vi "Get Intermediate Result.vi"(8 "error in (no error)":errorcluster, 11 "AverageCollector1D in":refnum<class "AverageCollector1D.lvclass">) -> (0 "error out":errorcluster, 2 "AbstractData.lvclass":refnum<class "AbstractData.lvclass">, 3 "AverageCollector1D out":refnum<class "AverageCollector1D.lvclass">)   [LabVIEW 2014, in "AverageCollector1D.lvclass"]
uses:
  AverageCollector1D.lvclass
  Framework/Model/Data/AbstractData/AbstractData.lvclass
  Framework/Collector/AbstractCollector/AbstractCollector.lvclass/AbstractCollector.ctl
  Framework/Model/Data/Data1D/Data1D.lvclass
  Framework/Collector/AbstractCollector/AbstractCollector.lvclass
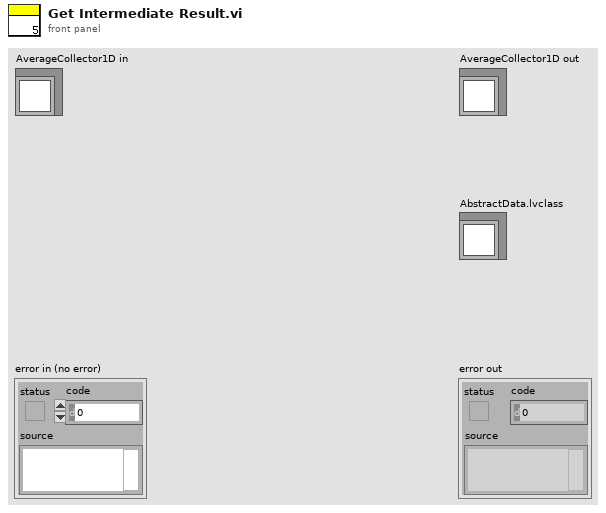
[diagram p1: front panel]
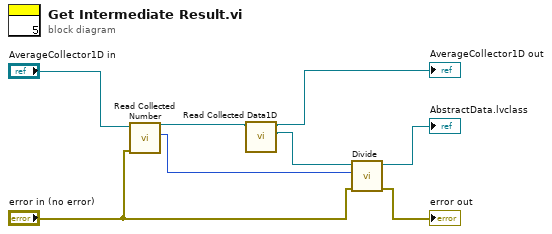
[diagram p0: block diagram]
diagram:
  n1 = call "Read Collected Number.vi"("error in (no error)"="error in (no error)", "AbstractCollector in"="AverageCollector1D in") -> ("collected"=w7:u32, "AbstractCollector out"=w4:refnum<class "AverageCollector1D.lvclass">)  [unwired: 7 in, 1 out]
  n2 = call-dynamic "Read Collected Data1D.vi"("AbstractCollector1D in"=w4) -> ("Collected Data"=w3:refnum<class "Data1D.lvclass">, "AbstractCollector1D out"=→"AverageCollector1D out":refnum<class "AverageCollector1D.lvclass">)  [unwired: 8 in, 1 out]
  n3 = call-dynamic "Divide.vi"("error in (no error)"="error in (no error)", "Divider"=w7, "Data1D in"=w3) -> ("error out"=→"error out":errorcluster, "Data1D out"=→"AbstractData.lvclass":refnum<class "Data1D.lvclass">)  [unwired: 7 in]
